vi "Shoulder Immediate.vi"(7 "Description":string, 8 "Command Info In":T1, 11 "Setpoint":dbl) -> (0 "Command Info Out":T1)   [LabVIEW 2018]
doc: "This template is useful for immediate subsystem actions that do not need deadband filtering\n\nBe sure to right-click and select New from Template and save with a new command name."
uses:
  <vilib>/Rock Robotics/WPI/Framework/Command Status Info.ctl
  <vilib>/Rock Robotics/WPI/Framework/Completion Status.ctl
  <vilib>/Rock Robotics/WPI/Framework/Completion Notifier.ctl
  Implementation/Shoulder Setpoints.ctl
  Implementation/Shoulder Operations.ctl
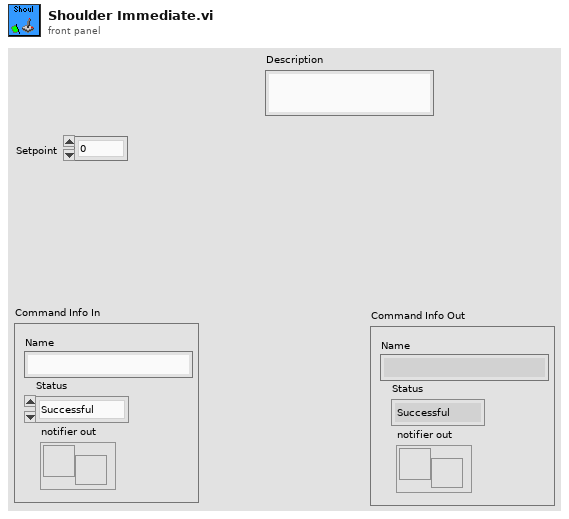
[diagram p1: front panel]
types:
  T1 = typedef "Command Status Info.ctl" = cluster{"Name":string, "Status":T2, "notifier out":T3}
  T2 = typedef "Completion Status.ctl" = enum16{"Successful", "Aborted", "Incomplete"}
  T3 = typedef "Completion Notifier.ctl" = refnum<notifier>
  T4 = typedef "Shoulder Setpoints.ctl" = cluster{"Operation":T5, "Setpoint":dbl}
  T5 = typedef "Shoulder Operations.ctl" = enum16{"Reserve", "Read Current", "Immediate"}
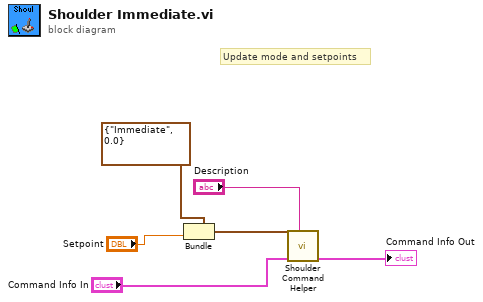
[diagram p0: block diagram]
diagram:
  # "Update mode and setpoints"
  n1 = Bundle(cluster=T4 {"Operation"=enum."Immediate", "Setpoint"=0.0} ("SubSystem Data"), "Setpoint"="Setpoint") -> (w2:T4)  [unwired: 1 in]
  n2 = call "Shoulder Command Helper.vi"("Description"="Description", "Command Info In"="Command Info In", "SubSystem Data"=w2) -> ("Command Info Out"=→"Command Info Out":T1)  [unwired: 6 in, 2 out]
